vi "Assert True.vi"(7 "Message (\"\")":string, 8 "error in (no error)":errorcluster, 10 "Condition":bool) -> (0 "error out":errorcluster)   [LabVIEW 2017, in "Transparent Assertions.lvlib"]
doc: "Asserts that a condition is <B>true</B>. Returns an error if the assertion fails, and optionally appends a custom message to the error."
uses:
  Transparent Assertions.lvlib
  IsTrue/IsTrue.lvclass
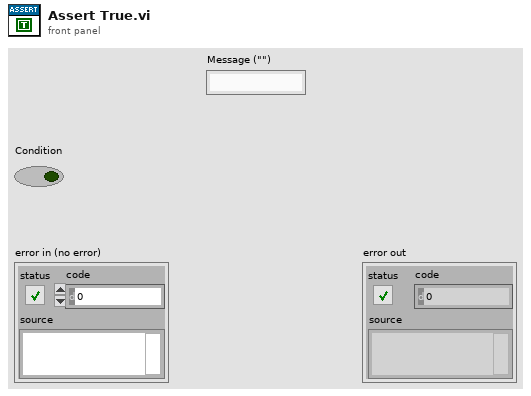
[diagram p1: front panel]
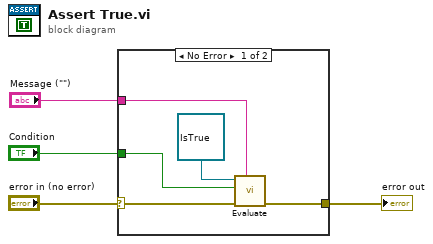
[diagram p0: block diagram]
diagram:
  n1 = case shown="No Error" "error in (no error)" {
    selector: "error in (no error)" -> [w8 w10]
    tunnel: "Condition" -> [w5 _]
    tunnel: [w7 w10] -> w2
    tunnel: "Message (\"\")" -> [w6 _]
    frame No Error {
      n2 = call-dynamic "Evaluate.vi"("Message (\"\")"=w6, "error in (no error)"=w8, "Actual"=w5, "Constraint in"=refnum<class "IsTrue.lvclass"> refnum ("IsTrue.lvclass")) -> ("error out"=w7:errorcluster)  [unwired: 6 in, 1 out]
    }
    frame Error {
    }
  }
  "error out" <- w2
